vi "KeyUp.vi"(9 "Virtual Key":u8(ring)=65) -> ()   [LabVIEW 2015]
doc: "Call the keybd_event function in user32.dll to generate an event corresponding to the key up action\nfor the desired key"
uses:
  user32.dll
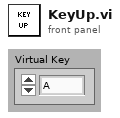
[diagram p1: front panel]
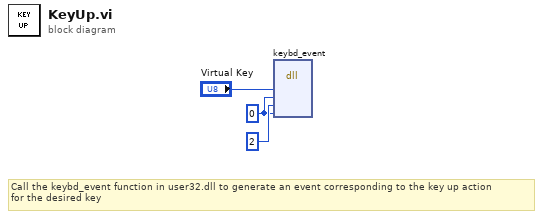
[diagram p0: block diagram]
diagram:
  w2 = u8 0 ("bScan")
  # "Call the keybd_event function in user32.dll to generate an event corresponding to the key up action\nfor the desired key"
  n1 = dll-call lib="user32.dll" fn="keybd_event"("bVk"="Virtual Key", "bScan"=w2, "dwFlags"=u32 2, "dwExtraInfo"=w2) -> ()  [unwired: 8 in, 2 out]
